vi "SwitchEditor.vi"(8 "error in (no error)":errorcluster, 10 "Length":enum16{"Long", "Short"}(ring)) -> (0 "error out":errorcluster)   [LabVIEW 2014]
uses:
  AutoMapBuilder/Controls/SwitchOp.ctl
  Libraries/Map Data Folder/Map Data.lvlib
panel:
  in  "SwitchOp":T1[](array[typedef])
  in  "Update":i32=1000
  in  "Stop":bool
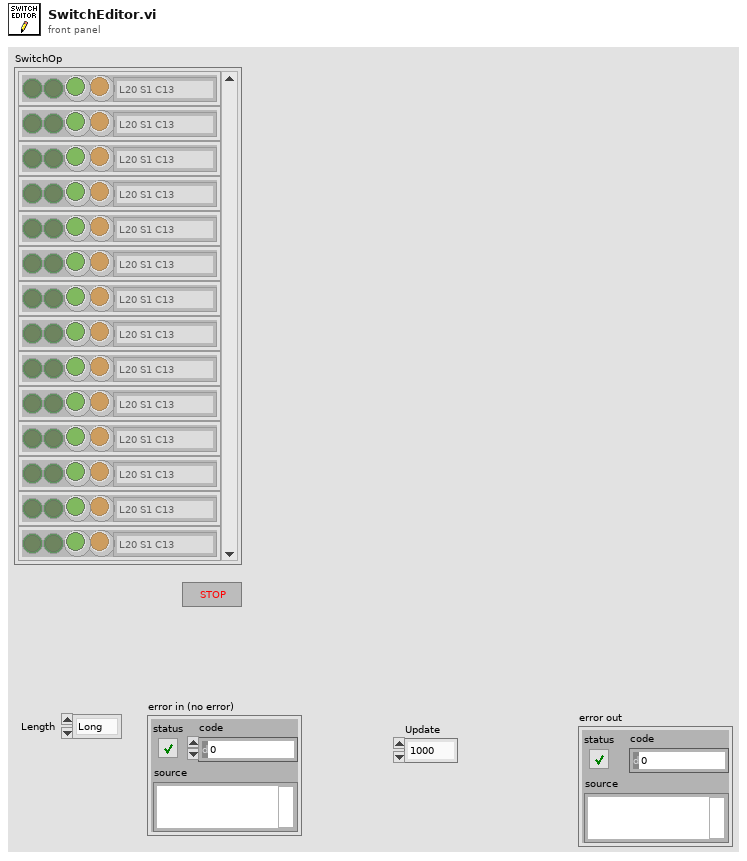
[diagram p1: front panel]
types:
  T1 = typedef "SwitchOp.ctl" = cluster{"Switch operational":bool, "Switch State":bool, "Manual Overide":bool, "Manual State":bool, "Switch\nPosition":cluster{"X":dbl, "Y":dbl, "Z":dbl}, "Index":i32, "Connection Index":i32, "Switch Index":i32, string}
  T2 = enum32{"Invalid", "Standard", "Closed", "Hidden", "Minimized", "Maximized"}
  T3 = typedef "Map Data.lvlib/All-Lines.ctl" = T4[]
  T4 = typedef "Map Data.lvlib/LineCluster.ctl" = cluster{"Line name":string, "Line array":cluster{"X":dbl, "Y":dbl, "Z":dbl}[], "Line connections":T5[]}
  T5 = typedef "Map Data.lvlib/LineConnection.ctl" = cluster{"Index":i32, "Switch Pos":cluster{"X":dbl, "Y":dbl, "Z":dbl}, "Switch operational":bool, "Switch State":bool, "Connection Index":i32, "Connection Pos":cluster{"X":dbl, "Y":dbl, "Z":dbl}, "LinePos Index":i32, "ConnectPos Index":i32, "Same direction?":bool, "Manual Overide":bool, "Manual State":bool}
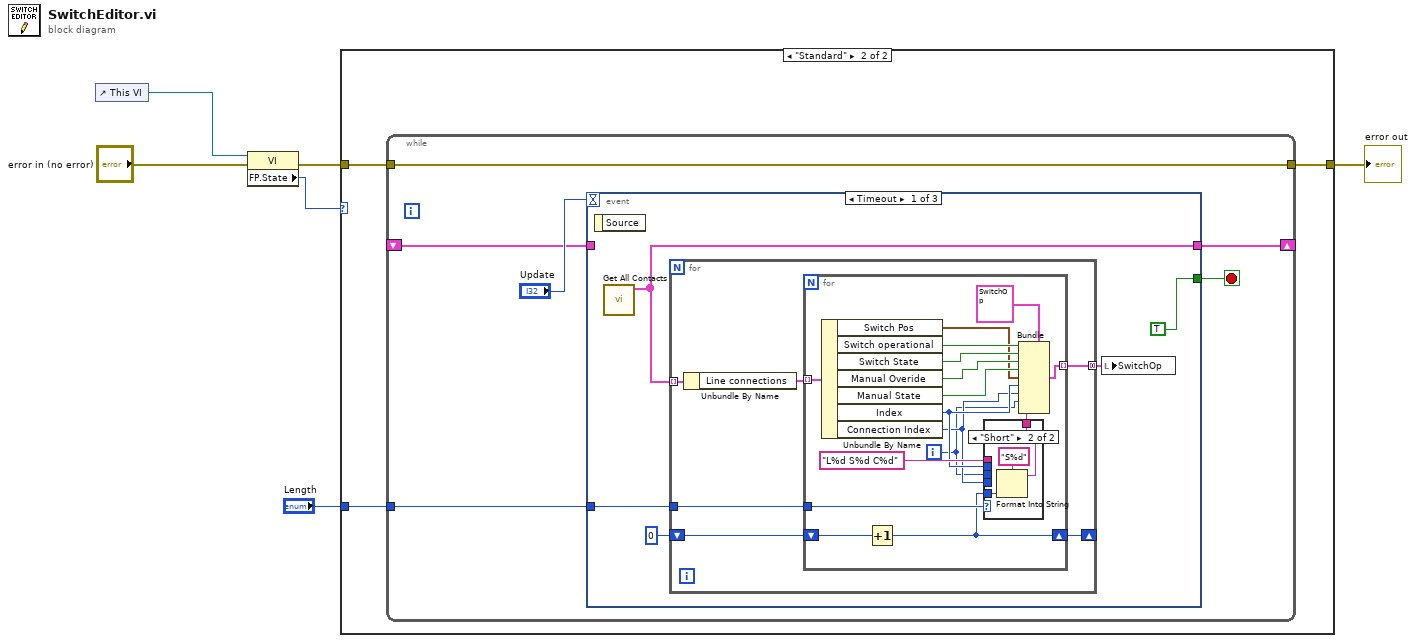
[diagram p0: block diagram]
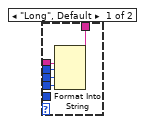
[diagram p3: hidden frame]
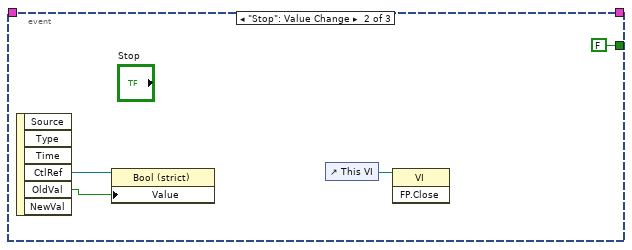
[diagram p4: hidden frame]
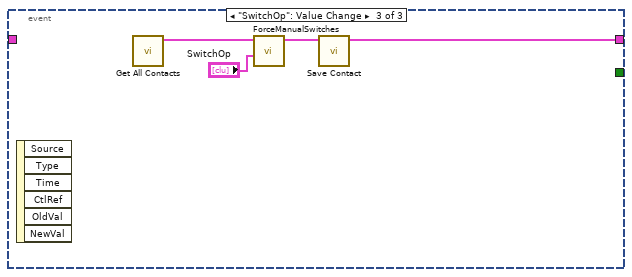
[diagram p5: hidden frame]
diagram:
  n1 = control-ref of="This VI"() -> (w5:refnum<vi>)
  n2 = property class="VI"(reference=w5, error in="error in (no error)") -> (error out=w4:errorcluster, "FP.State"=w2:T2)  [unwired: 1 out]
  n3 = case shown="\"Standard\"" w2 {
    tunnel: w4 -> [w7 w10]
    tunnel: [w7 w9] -> w3
    tunnel: "Length" -> [_ w8]
    frame "Invalid", Default {
    }
    frame "Standard" {
      n4 = while {
        shift-right: [w13] -> _
        shift-left: _ -> [w14]
        tunnel: w10 -> [w12]
        tunnel: [w12] -> w9
        tunnel: w8 -> [w11]
        stop <- w16 stop-if-true
        n5 = event shown="[0] Timeout" {
          selector: _ -> [_ _ _]
          dyn-events: _ -> [_ _ _]
          timeout: "Update" -> [_ _ _]
          tunnel: [TRUE FALSE _] -> w16
          tunnel: [w19 _ w56] -> w13
          tunnel: w14 -> [_ _ _]
          tunnel: w11 -> [w18 _ _]
          event Timeout {
            n6 = event-data() -> ()  [unwired: 1 in, 1 out]
            n7 = call "Get All Contacts.vi"() -> ("All Lines out"=w19:T3)  [unwired: 9 in, 2 out]
            n8 = for {
              tunnel: w19 -> [w27] mode=indexing
              tunnel: [w25] -> w20 mode=concatenating
              tunnel: w18 -> [w24]
              shift-right: [w22] -> _
              shift-left: 0 -> [w23]
              n9 = Unbundle By Name(w27) -> ("Line connections"=w26:T5[])
              n10 = for {
                tunnel: w26 -> [w43] mode=indexing
                tunnel: [w41] -> w25 mode=indexing
                tunnel: w24 -> [w30]
                shift-right: [w28] -> w22
                shift-left: w23 -> [w29]
                i -> [w31]
                n11 = Unbundle By Name(w43) -> ("Switch Pos"=w35:cluster{"X":dbl, "Y":dbl, "Z":dbl}, "Switch operational"=w39:bool, "Switch State"=w38:bool, "Manual Overide"=w37:bool, "Manual State"=w36:bool, "Index"=w34:i32, "Connection Index"=w33:i32)
                n12 = Increment(x=w29) -> (x+1=w28:i32)
                n13 = case shown="\"Short\"" w30 {
                  tunnel: "L%d S%d C%d" ("format string") -> [w48 _]
                  tunnel: w34 -> [w47 _]
                  tunnel: w33 -> [w46 _]
                  tunnel: [w45 w50] -> w32
                  tunnel: w31 -> [w44 _]
                  tunnel: w28 -> [_ w49]
                  frame "Long", Default {
                    n14 = Format Into String(format string=w48, w47, w44, w46) -> (resulting string=w45:string)  [unwired: 2 in, 1 out]
                  }
                  frame "Short" {
                    n15 = Format Into String(format string="S%d", w49) -> (resulting string=w50:string)  [unwired: 2 in, 1 out]
                  }
                }
                n16 = Bundle(cluster=T1 {"Switch operational"=FALSE, "Switch State"=FALSE, "Manual Overide"=FALSE, "Manual State"=FALSE, "Switch\nPosition"={"X"=1401.4972181059047, "Y"=55.368, "Z"=5623.149736695605}, "Index"=0, "Connection Index"=3, "Switch Index"=0, "L0 S0 C3"}, "Switch operational"=w39, "Switch State"=w38, "Manual Overide"=w37, "Manual State"=w36, "Switch\nPosition"=w35, "Index"=w34, "Connection Index"=w33, "Switch Index"=w31, w32) -> (w41:T1)
              }
            }
            n17 = local write "SwitchOp"(w20) -> ()
          }
          event "Stop": Value Change {
            n18 = event-data() -> ("CtlRef"=w53:refnum<vi>, "OldVal"=w52:bool)  [unwired: 1 in, 4 out]
            n19 = property class="Bool (strict)"(reference=w53, "Value"=w52) -> ()  [unwired: 1 in, 2 out]
            n20 = control-ref of="This VI"() -> (w55:refnum<vi>)
            n21 = invoke class="VI" method="FP.Close"(reference=w55) -> ()  [unwired: 2 in, 3 out]
          }
          event "SwitchOp": Value Change {
            n22 = event-data() -> ()  [unwired: 1 in, 6 out]
            n23 = call "Get All Contacts.vi"() -> ("All Lines out"=w58:T3)  [unwired: 9 in, 2 out]
            n24 = call "ForceManualSwitches.vi"("Switch Op"="SwitchOp", "output array 2"=w58) -> ("output array 3"=w57:T3)  [unwired: 9 in]
            n25 = call "Save Contact.vi"("All Lines"=w57) -> ("All Lines out"=w56:T3)  [unwired: 9 in, 1 out]
          }
        }
      }
    }
  }
  "error out" <- w3
